vi "TimeTag_LSW_edits_Sept6.vi"() -> ()   [LabVIEW 2015]
doc: "This sample project is built upon the standard state machine template and shows how you could create an application that acquires, analyzes, and presents data. It includes functionality for presenting configuration dialogs, preserving settings between executions, loading and saving data, as well as exporting graph images and text files.\n\nIt is most appropriate for data that is acquired instantly as it does not allow for screen updates mid acquisition nor does it allow for continuous streaming to disk."
uses:
  <vilib>/ptbypt/NI_PtbyPt.lvlib
panel:
  out "Ch4 100sec avg":dbl
  out "Ch2 100 sec avg":dbl
  out "real coin cps 100 pt\n avg":dbl
  out "all coin cps":dbl
  out "real coin cps":dbl
  out "random coin cps":dbl
  out "Real coin cps":dbl(graph)
  out "total coin/sec - total random coin/sec":dbl
  out "total random coincidences/sec":dbl
  out "Total Coin per sec":dbl
  out "Ch2/4 coin/sec":dbl(graph)
  out "Ch2/4 Total Coincidences":dbl
  out "Channel 2 CPS":dbl(graph)
  out "Channel 4 CPS":dbl(graph)
  out "Total Ch2 CPS":dbl
  out "Total Ch4 CPS":dbl
  in  "Averaging":dbl=10.0
  in  "Runs":dbl=100.0
  in  "Pulse TTL 2":bool
  in  "Pulse TTL 1":bool
  in  "Toggle\nTTL 2":bool
  in  "Toggle\nTTL 1":bool
  out "Total Starts":dbl
  in  "Record data":bool
  out "Initial time":dbl
  out "Elapsed time (s)":dbl
  out "FPGA_Run Status":dbl
  out "USB_Open Status":dbl
  out "Channel 4 Total\nCounts":dbl
  out "Channel 3 Total\nCounts":dbl
  out "Channel 2 Total\nCounts":dbl
  out "Channel 1 Total\nCounts":dbl
  in  "File Name":string="C:\\FPGA\\test.txt"
  out "?":dbl
  out "?":dbl
  out "?":dbl
  out "?":dbl
  out "stats":i64[](array[numeric])
  in  "Stop":bool
  out "Channel 4 CPS":dbl(knob) scale=0.0..2000000.0
  out "Channel 3 CPS":dbl(knob) scale=0.0..600.0
  out "Channel 2 CPS":dbl(knob) scale=0.0..700.0
  out "Channel 1 CPS":dbl(knob) scale=0.0..600.0
  # "Starts"
  # "Channel 1"
  # "Channel 2"
  # "Channel 3"
  # "Channel 4"
  # "Coincidence Channels 1 & 2"
  # "Coincidence Channels 1 & 3"
  # "Coincidence Channels 1 & 4"
  # "Coincidence Channels 2 & 3"
  # "Coincidence Channels 2 & 4"
  # "Coincidence Channels 3 & 4"
  # "Coincidence Channels 1 & 2 & 3"
  # "Coincidence Channels 1 & 2 & 4"
  # "Coincidence Channels 1 & 3 & 4"
  # "Coincidence Channels 2 & 3 & 4"
  # "C:\\FPGA_Lauren"
  # "Coincidence Channels 1 & 2 & 3 & 4"
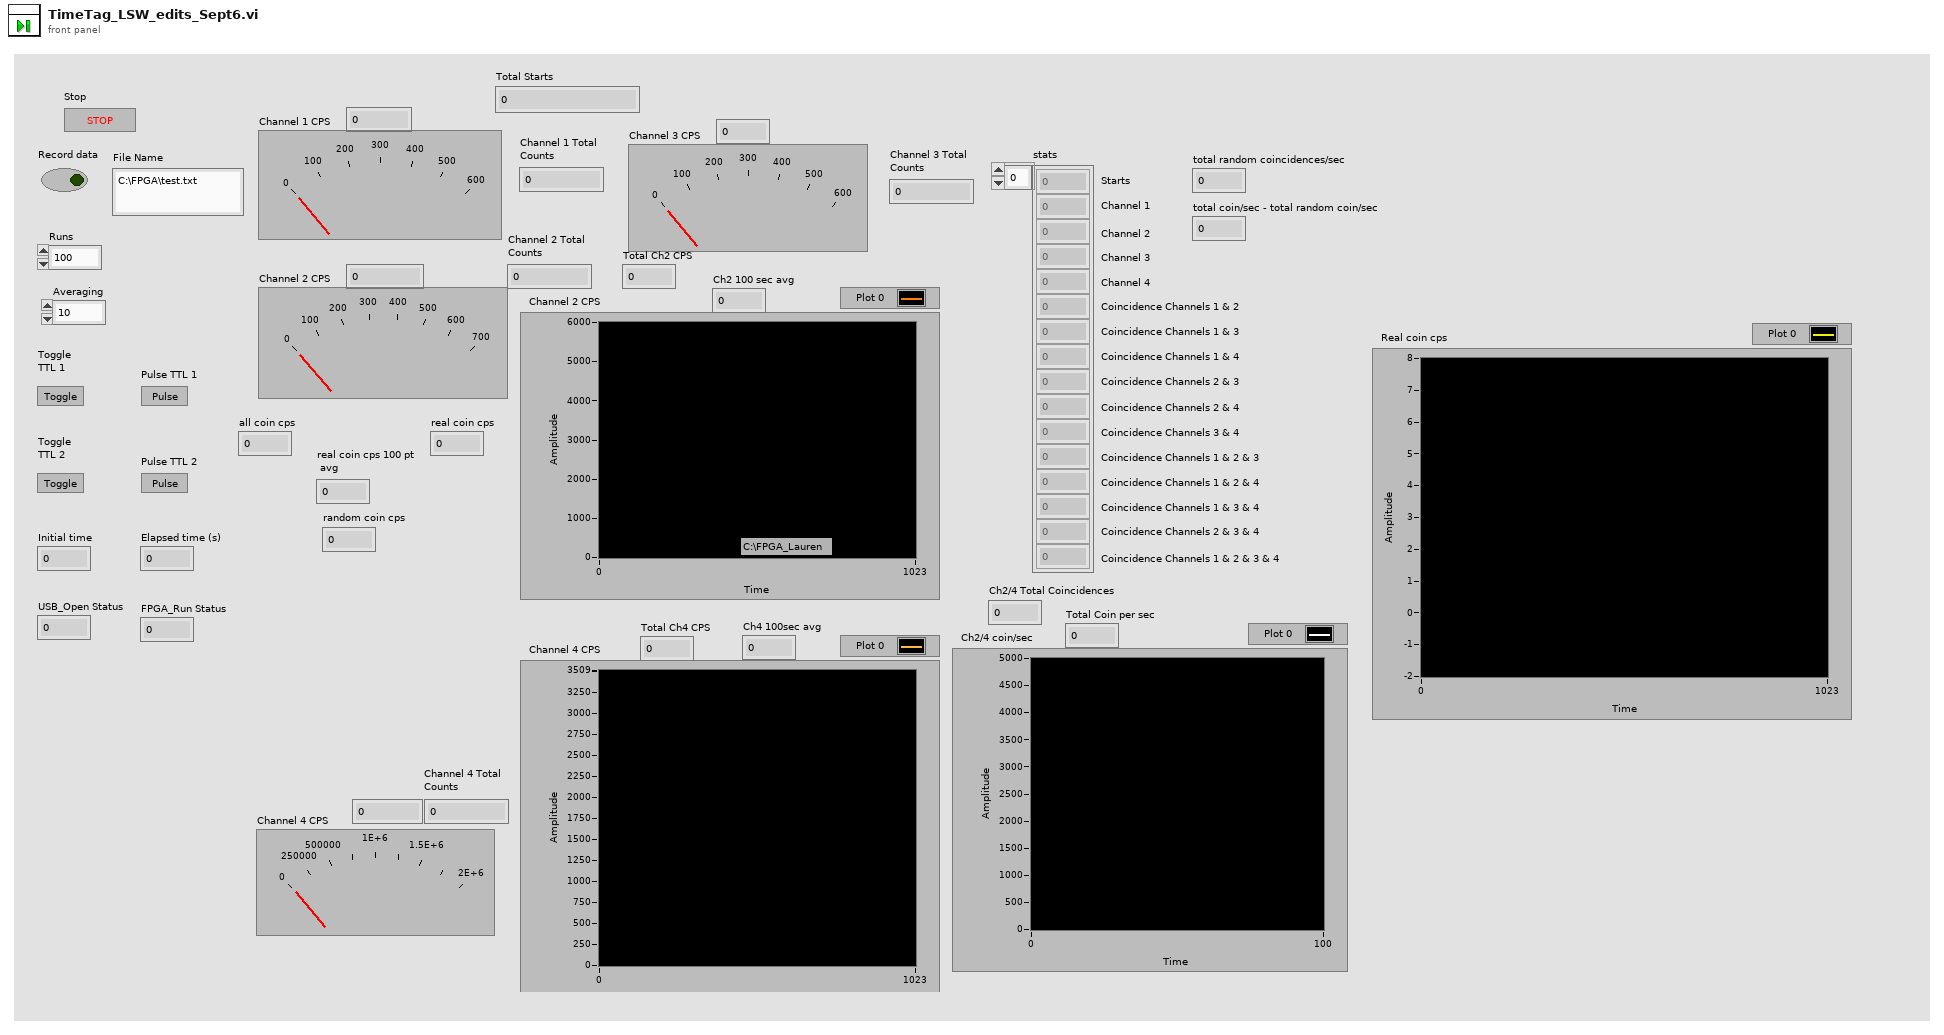
[diagram p1: front panel]
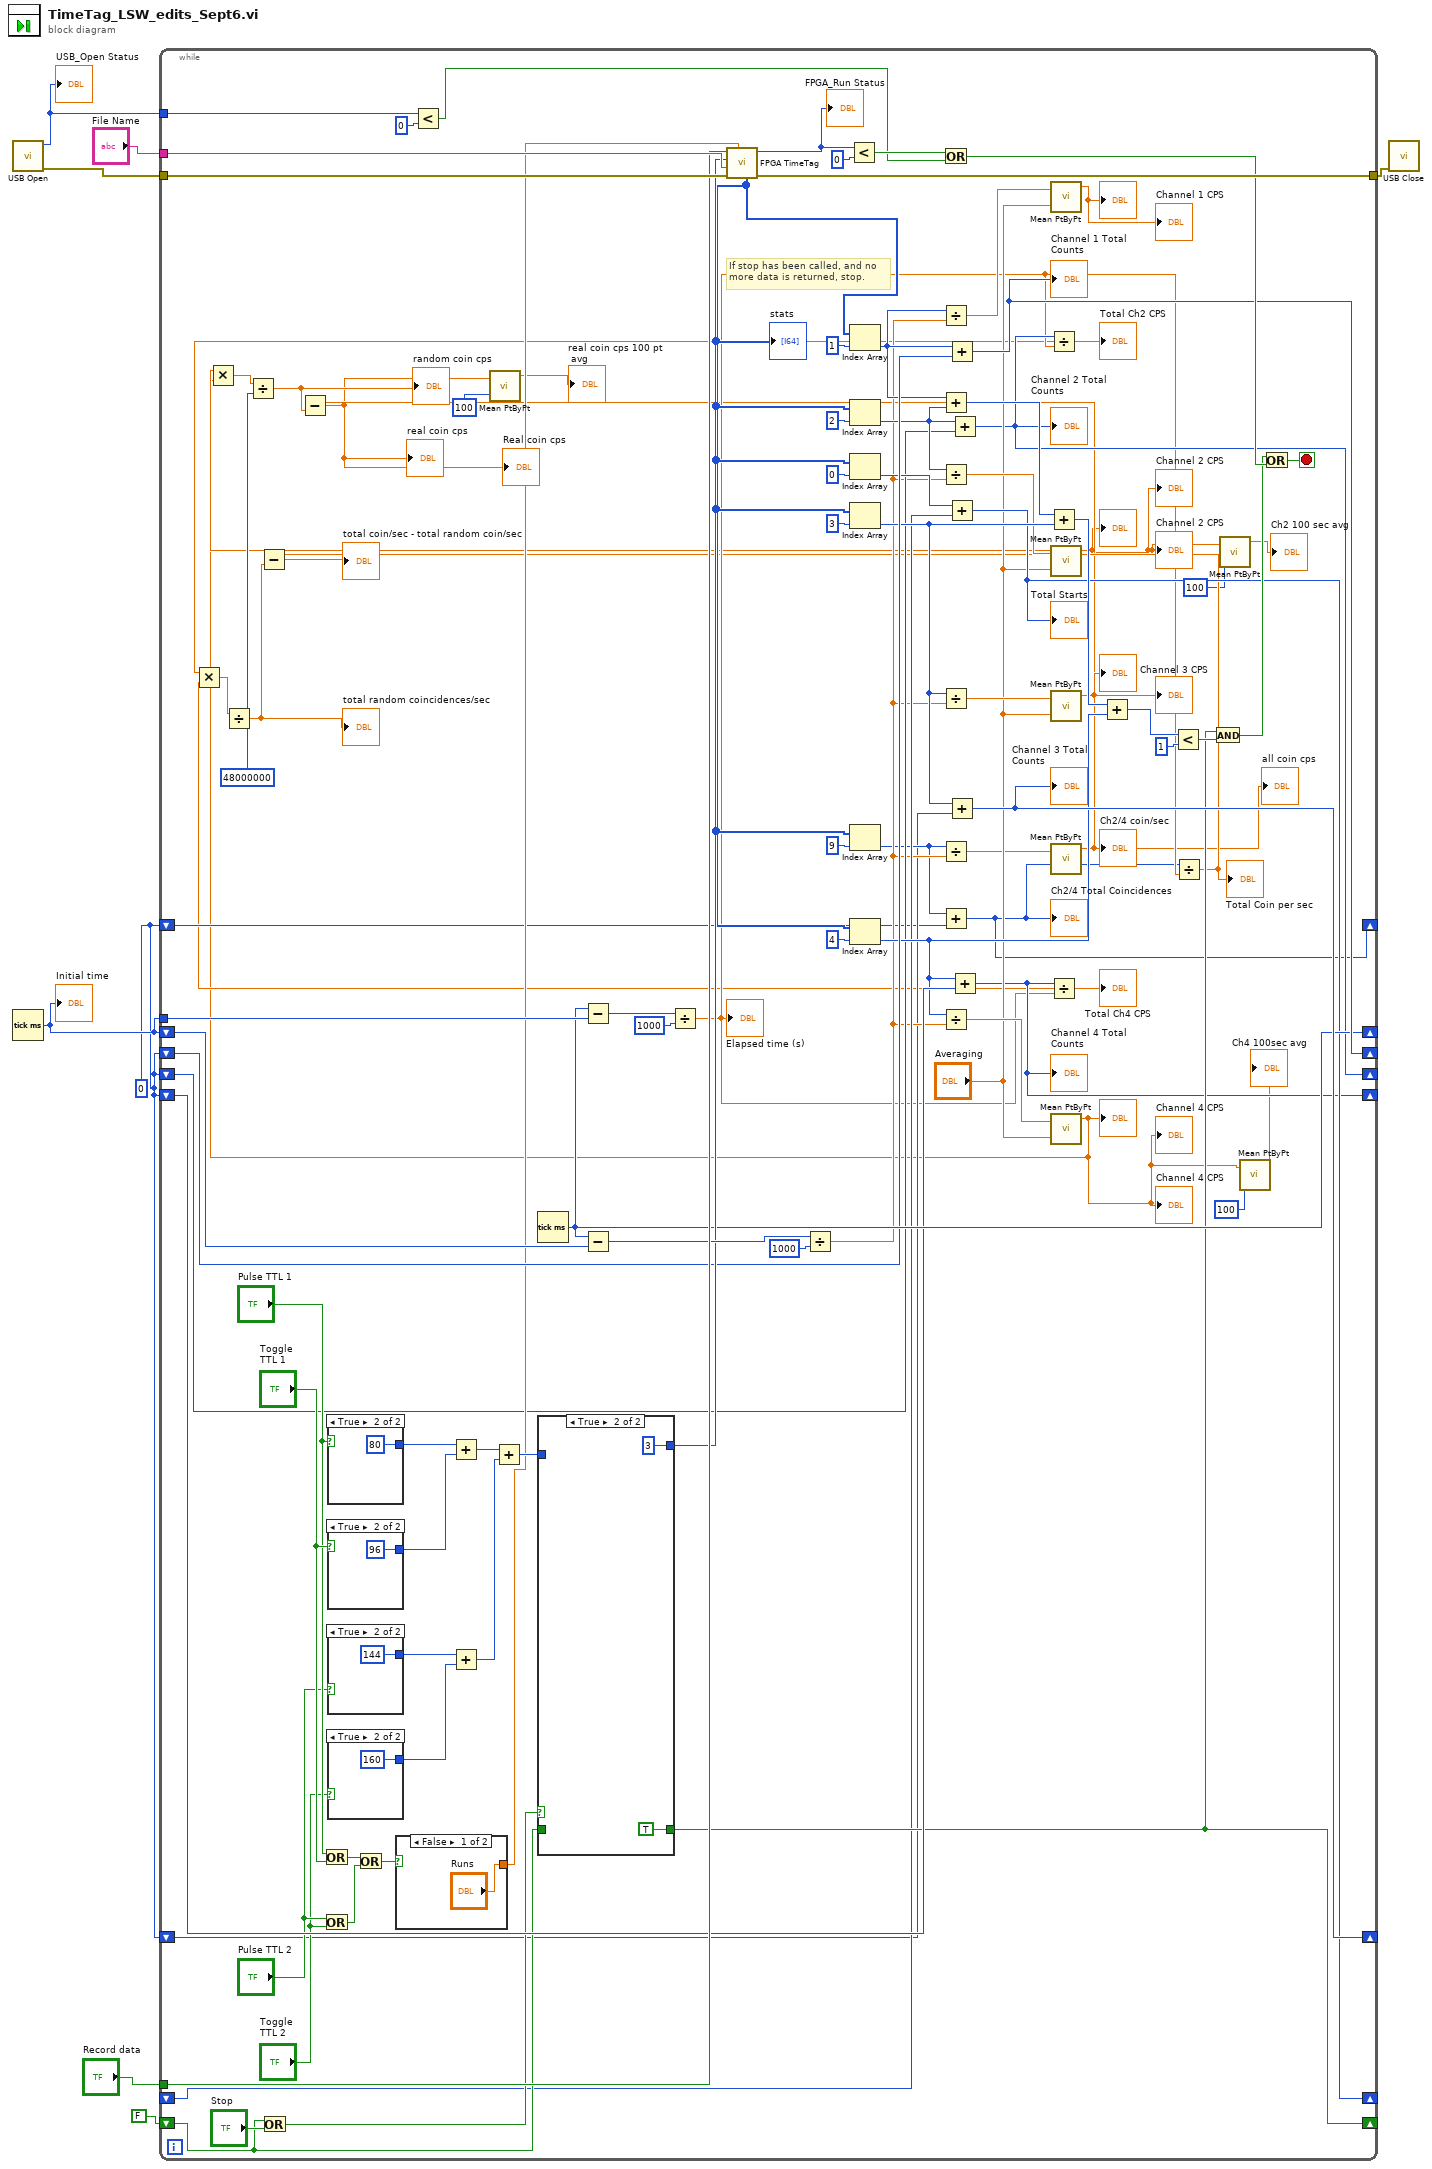
[diagram p0: block diagram]
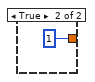
[diagram p2: hidden frame]
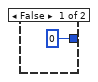
[diagram p3: hidden frame]
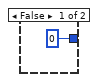
[diagram p4: hidden frame]
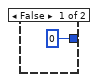
[diagram p5: hidden frame]
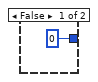
[diagram p6: hidden frame]
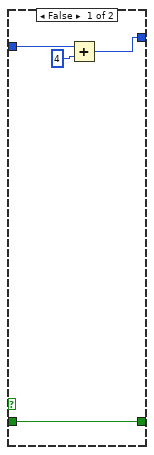
[diagram p7: hidden frame]
diagram:
  w1 = 0
  n1 = call "USB Open.vi"() -> ("error out"=w6:errorcluster, "function return"=w3:i32)  [unwired: 10 in]
  "USB_Open Status" <- w3
  n2 = Tick Count (ms)() -> (millisecond timer value=w4:u32)
  "Initial time" <- w4
  n3 = while {
    tunnel: w4 -> [w107]
    shift-right: [w85] -> _
    shift-left: w1 -> [w81]
    shift-right: [w39] -> _
    shift-left: w1 -> [w35]
    shift-right: [w84] -> _
    shift-left: w1 -> [w31]
    shift-right: [w40] -> _
    shift-left: w1 -> [w80]
    tunnel: w6 -> [w97]
    tunnel: [w98] -> w5
    tunnel: "Record data" -> [w95]
    tunnel: "File Name" -> [w96]
    shift-right: [w82] -> _
    shift-left: w4 -> [w93]
    tunnel: w3 -> [w89]
    shift-right: [w69] -> _
    shift-left: FALSE -> [w66]
    shift-right: [w62] -> _
    shift-left: _ -> [w63]
    shift-right: [w28] -> _
    shift-left: w1 -> [w30]
    stop <- w99 stop-if-true
    w22 = 48000000
    # "If stop has been called, and no\nmore data is returned, stop."
    n4 = Or(x=w66, y="Stop") -> (x .or. y?=w68:bool)
    n5 = Or(x="Pulse TTL 1", y="Toggle\nTTL 1") -> (x .or. y?=w53:bool)
    n6 = Or(x="Pulse TTL 2", y="Toggle\nTTL 2") -> (x .or. y?=w54:bool)
    n7 = case shown="True" "Pulse TTL 1" {
      tunnel: [0 80] -> w61
      frame False {
      }
      frame True {
      }
    }
    n8 = case shown="True" "Toggle\nTTL 1" {
      tunnel: [0 96] -> w60
      frame False {
      }
      frame True {
      }
    }
    n9 = case shown="True" "Pulse TTL 2" {
      tunnel: [0 144] -> w57
      frame False {
      }
      frame True {
      }
    }
    n10 = case shown="True" "Toggle\nTTL 2" {
      tunnel: [0 160] -> w58
      frame False {
      }
      frame True {
      }
    }
    n11 = Or(x=w53, y=w54) -> (x .or. y?=w55:bool)
    n12 = case shown="False" w55 {
      tunnel: ["Runs" 1] -> w51
      frame False {
      }
      frame True {
      }
    }
    n13 = Less?(x=w89, y=0) -> (x < y?=w87:bool)
    n14 = Add(x=w61, y=w60) -> (x+y=w59:i32)
    n15 = Add(x=w57, y=w58) -> (x+y=w56:i32)
    n16 = Add(x=w59, y=w56) -> (x+y=w52:i32)
    n17 = Tick Count (ms)() -> (millisecond timer value=w82:u32)
    n18 = case shown="True" w68 {
      tunnel: [w119 3] -> w83
      tunnel: [w121 TRUE] -> w69
      tunnel: w66 -> [w121 _]
      tunnel: w52 -> [w118 _]
      frame False {
        n19 = Add(x=w118, y=4) -> (x+y=w119:i32)
      }
      frame True {
      }
    }
    n20 = Subtract(x=w82, y=w107) -> (x-y=w106:u32)
    n21 = Subtract(x=w82, y=w93) -> (x-y=w92:u32)
    n22 = Divide(x=w106, y=1000) -> (x/y=w29:dbl)
    "Elapsed time (s)" <- w29
    n23 = call "FPGA TimeTag.vi"("runs"=w51, "error in (no error)"=w97, "fileName"=w96, "fpgaCommand"=w83, "saveData"=w95) -> ("error out"=w98:errorcluster, "function return"=w94:i32, "stats"=w37:i64[])  [unwired: 4 in]
    "stats" <- w37
    "FPGA_Run Status" <- w94
    n24 = Divide(x=w92, y=1000) -> (x/y=w34:dbl)
    n25 = Less?(x=w94, y=0) -> (x < y?=w88:bool)
    n26 = Index Array(array=w37, index=1) -> (element=w72:i64)
    n27 = Index Array(array=w37, index=2) -> (element=w79:i64)
    n28 = Index Array(array=w37, index=0) -> (element=w64:i64)
    n29 = Index Array(array=w37, index=3) -> (element=w75:i64)
    n30 = Index Array(array=w37, index=9) -> (element=w32:i64)
    n31 = Index Array(array=w37, index=4) -> (element=w76:i64)
    n32 = Or(x=w88, y=w87) -> (x .or. y?=w86:bool)
    n33 = Divide(x=w72, y=w34) -> (x/y=w46:dbl)
    n34 = Add(x=w72, y=w79) -> (x+y=w74:i64)
    n35 = Divide(x=w79, y=w34) -> (x/y=w45:dbl)
    n36 = Divide(x=w75, y=w34) -> (x/y=w44:dbl)
    n37 = Divide(x=w32, y=w34) -> (x/y=w33:dbl)
    n38 = Add(x=w32, y=w30) -> (x+y=w28:i64)
    "Ch2/4 Total Coincidences" <- w28
    n39 = Divide(x=w76, y=w34) -> (x/y=w42:dbl)
    n40 = Add(x=w72, y=w81) -> (x+y=w85:i64)
    "Channel 1 Total\nCounts" <- w85
    n41 = Add(x=w64, y=w63) -> (x+y=w62:i64)
    "Total Starts" <- w62
    n42 = Add(x=w75, y=w31) -> (x+y=w84:i64)
    "Channel 3 Total\nCounts" <- w84
    n43 = Add(x=w79, y=w35) -> (x+y=w39:i64)
    "Channel 2 Total\nCounts" <- w39
    n44 = Add(x=w76, y=w80) -> (x+y=w40:i64)
    "Channel 4 Total\nCounts" <- w40
    n45 = Divide(x=w39, y=w29) -> (x/y=w25:dbl)
    "Total Ch2 CPS" <- w25
    n46 = Add(x=w74, y=w75) -> (x+y=w78:i64)
    n47 = Divide(x=w40, y=w29) -> (x/y=w24:dbl)
    "Total Ch4 CPS" <- w24
    n48 = Multiply(x=w25, y=w24) -> (x*y=w23:dbl)
    n49 = Divide(x=w23, y=w22) -> (x/y=w26:dbl)
    "total random coincidences/sec" <- w26
    n50 = call <vilib>:"Mean PtByPt.vi"("x"=w46, "sample length"="Averaging") -> ("mean"=→"Channel 1 CPS" →"?":dbl)  [unwired: 2 in, 1 out]
    n51 = call <vilib>:"Mean PtByPt.vi"("x"=w45, "sample length"="Averaging") -> ("mean"=w14:dbl)  [unwired: 2 in, 1 out]
    "Channel 2 CPS" <- w14
    "?" <- w14
    "Channel 2 CPS" <- w14
    n52 = call <vilib>:"Mean PtByPt.vi"("x"=w44, "sample length"="Averaging") -> ("mean"=→"Channel 3 CPS" →"?":dbl)  [unwired: 2 in, 1 out]
    n53 = call <vilib>:"Mean PtByPt.vi"("x"=w33) -> ("mean"=w18:dbl)  [unwired: 3 in, 1 out]
    "Ch2/4 coin/sec" <- w18
    "all coin cps" <- w18
    n54 = call <vilib>:"Mean PtByPt.vi"("x"=w42, "sample length"="Averaging") -> ("mean"=w11:dbl)  [unwired: 2 in, 1 out]
    "Channel 4 CPS" <- w11
    "?" <- w11
    "Channel 4 CPS" <- w11
    n55 = Multiply(x=w14, y=w11) -> (x*y=w21:dbl)
    n56 = Divide(x=w21, y=w22) -> (x/y=w20:dbl)
    "random coin cps" <- w20
    n57 = Subtract(x=w18, y=w20) -> (x-y=w17:dbl)
    "Real coin cps" <- w17
    "real coin cps" <- w17
    n58 = call <vilib>:"Mean PtByPt.vi"("x"=w17, "sample length"=100) -> ("mean"=→"real coin cps 100 pt\n avg":dbl)  [unwired: 2 in, 1 out]
    n59 = Add(x=w78, y=w76) -> (x+y=w77:i64)
    n60 = Less?(x=w77, y=1) -> (x < y?=w71:bool)
    n61 = Divide(x=w28, y=w29) -> (x/y=w27:dbl)
    "Total Coin per sec" <- w27
    n62 = Subtract(x=w27, y=w26) -> (x-y=→"total coin/sec - total random coin/sec":dbl)
    n63 = And(x=w69, y=w71) -> (x .and. y?=w70:bool)
    n64 = call <vilib>:"Mean PtByPt.vi"("x"=w14, "sample length"=100) -> ("mean"=→"Ch2 100 sec avg":dbl)  [unwired: 2 in, 1 out]
    n65 = call <vilib>:"Mean PtByPt.vi"("x"=w11, "sample length"=100) -> ("mean"=→"Ch4 100sec avg":dbl)  [unwired: 2 in, 1 out]
    n66 = Or(x=w70, y=w86) -> (x .or. y?=w99:bool)
  }
  n67 = call "USB Close.vi"("error in (no error)"=w5) -> ()  [unwired: 9 in, 2 out]
